vi "Msg To Nested.vi"(8 "Alias":string, 9 "Priority Msg?":bool, 10 "Msg":refnum<class "Msg Strategy.lvclass">, 11 "Self Actor in":refnum<class "Self Actor.lvclass">) -> (0 "error out":errorcluster)   [LabVIEW 2021, in "jettl.lvlib" / "Self Actor.lvclass"]
uses:
  Self Actor.lvclass
  Msg Strategy/Msg Strategy.lvclass
  Self Actor.lvclass/Self Actor.ctl
  jettl.lvlib
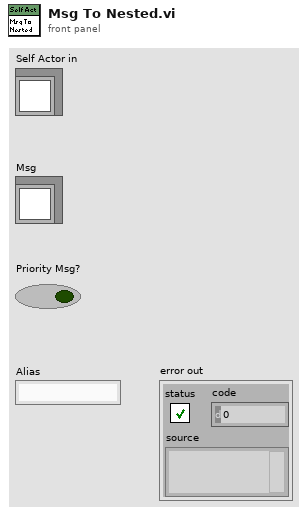
[diagram p1: front panel]
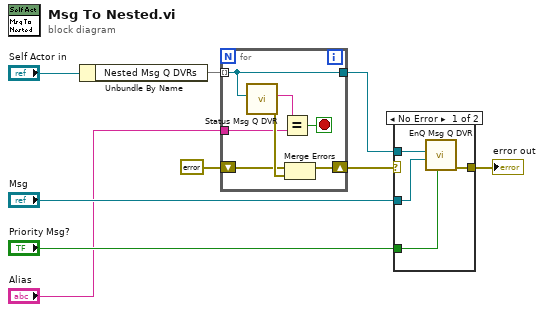
[diagram p0: block diagram]
diagram:
  n1 = Unbundle By Name("Self Actor in") -> ("Nested Msg Q DVRs"=w6:set{refnum<data-value>})
  n2 = for {
    tunnel: w6 -> [w16] mode=indexing
    tunnel: [w16] -> w1
    tunnel: "Alias" -> [w10]
    shift-right: [w11] -> w2
    shift-left: errorcluster {"status"=FALSE, "code"=0, "source"=""} ("error IO") -> [w12]
    stop <- w13 stop-if-true
    n3 = call "Status Msg Q DVR.vi"("Msg Q DVR"=w16) -> ("error out"=w14:errorcluster, "Msg Q DVR Alias"=w15:string)  [unwired: 9 in]
    n4 = Equal?(x=w15, y=w10) -> (x = y?=w13:bool)
    n5 = Merge Errors(w12, w14) -> (w11:errorcluster)
  }
  n6 = case shown="No Error" w2 {
    selector: w2 -> [_ w21]
    tunnel: [w20 w21] -> w7
    tunnel: "Msg" -> [w19 _]
    tunnel: "Priority Msg?" -> [w18 _]
    tunnel: w1 -> [w17 _]
    frame No Error {
      n7 = call "EnQ Msg Q DVR.vi"("Priority Msg?"=w18, "Msg"=w19, "Msg Q DVR"=w17) -> ("error out"=w20:errorcluster)  [unwired: 8 in]
    }
    frame Error {
    }
  }
  "error out" <- w7
